vi "SR430.get bin width.vi"(0 "i ref in":refnum<vi>, 5 "error in (no error)":errorcluster) -> (14 "i ref out":refnum<vi>, 16 "binWidth [us]":dbl format="%.3f", 19 "error out":errorcluster)   [LabVIEW 2014, in "SR430.lvlib"]
doc: "reads the width of the bin from the unit."
uses:
  SR430.lvlib
  CSCore/CSApplicationBaseClasses/MCSBase/MCSBase.directionType.ctl
  CSCore/CSApplicationBaseClasses/MCSBase/MCSBase.serviceType.ctl
  CSlibraries/UtilityLib/UtilityLib.valueStatus.ctl
  CSCore/CSSystem/CoreDefs/CoreDefs.error_type.ctl
  CSinstr.lib/Sr430/SR430Driver.lvlib
  CSCore/CSSystem/CoreLib/CoreLib.lvlib
  CSCore/CSApplicationBaseClasses/MCSBase/MCSBase.lvlib
  CSlibraries/UtilityLib/UtilityLib.lvlib
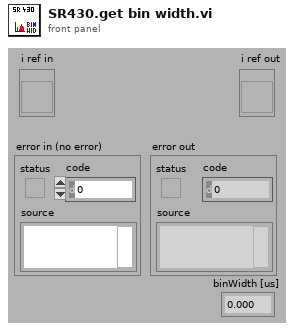
[diagram p1: front panel]
types:
  T1 = typedef "UtilityLib.lvlib/UtilityLib.valueStatus.ctl" = enum16{"no info available", "stand by/off", "on", "warning", "alarm/malfunction", "not implemented", "user action required", "important information", "system default", "control default", "indicator default", "button default"}
  T2 = typedef "MCSBase.lvlib/MCSBase.serviceType.ctl" = enum16{"counts", "totalCounts", "binWidth", "nOfBins", "nOfRecords", "status", "discrLevel", "discrSlope", "triggerLevel", "triggerSlope"}
  T3 = typedef "MCSBase.lvlib/MCSBase.directionType.ctl" = enum16{"unknown", "update actual value", "update nominal value", "update both"}
  T4 = typedef "CoreDefs.error_type.ctl" = enum16{"no error", "can't load process", "can't unload process", "process does not exist", "can't install process", "can't remove process", "unknown function", "time out", "can't execute function", "duplicate queue name", "super not found", "caller queue invalid", "can't ping process", "unknown error", "VISA Error", "VISA timeout", "GPIB timeout", "GPIB error", "communication error", "data type mismatch", "can't read data from OPC server", "can't write data to OPC server", "OET error", "function not implemented", "process already exists", "invalid Shared Variable name", "error writing Shared Variable", "error reading Shared Variable", "invalid client name", "corrupt database", "unknown class", "call not authorized", "parameter out of range", "OET timeout: can't get data to modify", "invalid queue name", "requested operation incompatible with current state", "event undefined", "event disabled", "state undefined", "caller is not a friend", "EventBuilder: bad eventID", "EventBuilder: no DAQ devices", "a thread must not stop itself", "UNUSED ELEMENT4", "DiscArchiver: eventData incomplete", "DiscArchiver: eventData does not belong to run", "DiscArchiver: can't open file", "DiscArchiver: can't write to file", "DiscArchiver: available disc space low", "can't acquire semaphore", "error reading data from database", "notifier object is not existing", "can't register process", "can't unregister process", "illegal event type", "object disabled", "object already exists", "can't change state", "Instrument not found", "no connection to remote node", "invalid reference", "N/A", "UNUSED ELEMENT 1", "element not found", "illegal TCP/IP connection detected", "object does not exist", "invalid access ID", "unknown CS system", "invalid privilige", "unsupported data type", "unsupported server type", "IO server already exists", "Shared Variable already exists"}
  T5 = typedef "SR430Driver.lvlib/SR430_VISA Control.ctl" = cluster{"VISA resource name":refnum<visa-resource-name>}
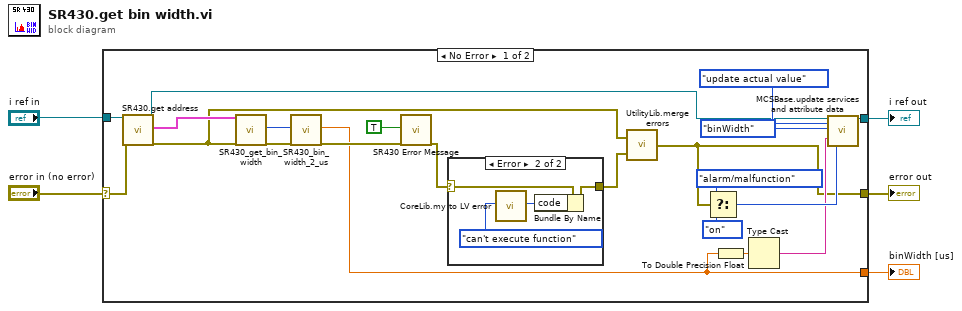
[diagram p0: block diagram]
diagram:
  n1 = case shown="No Error" "error in (no error)" {
    selector: "error in (no error)" -> [w17 w33]
    tunnel: "i ref in" -> [w26 w32]
    tunnel: [w6 w33] -> w4
    tunnel: [w8 w32] -> w3
    tunnel: [w7 _] -> w2
    frame No Error {
      n2 = call "SR430.get address.vi"("i ref in"=w26, "error in (no error)"=w17) -> ("i ref out"=w9:refnum<vi>, "address"=w25:T5, "error out"=w24:errorcluster)  [unwired: 15 in]
      n3 = call "SR430_get_bin_width.vi"("address"=w25, "error in (no error)"=w24) -> ("bin width"=w21:i32, "error out"=w22:errorcluster)  [unwired: 15 in, 1 out]
      n4 = call "SR430_bin_width_2_us.vi"("bin width"=w21, "error in (no error)"=w22) -> ("binWidth [us]"=w7:dbl, "error out"=w20:errorcluster)  [unwired: 15 in, 1 out]
      n5 = call "SR430 Error Message.vi"("addMessageToSource"=TRUE ("add message to source"), "error in (no error)"=w20) -> ("error out"=w23:errorcluster)  [unwired: 14 in, 3 out]
      n6 = case shown="Error" w23 {
        selector: w23 -> [w27 w31]
        tunnel: [w27 w28] -> w18
        frame No Error {
        }
        frame Error {
          n7 = call "CoreLib.my to LV error.vi"("ErrorTypes"=CoreDefs.error_type."can't execute function") -> ("LV error code"=w30:i32)  [unwired: 17 in, 1 out]
          n8 = Bundle By Name(cluster=w31, "code"=w30) -> (w28:errorcluster)
        }
      }
      n9 = call "UtilityLib.merge errors.vi"("error2 (no error)"=w18, "error1 (no error)"=w24) -> ("error out"=w6:errorcluster)
      n10 = Select(t=UtilityLib.valueStatus."alarm/malfunction" ("quality"), s=w6, f=UtilityLib.valueStatus."on") -> (s? t:f=w12:T1)
      n11 = To Double Precision Float(number=w7) -> (double precision float=w10:dbl)
      n12 = Type Cast(x=w10) -> (*(type *) &x=w11:string)  [unwired: 1 in]
      n13 = call "MCSBase.update services and attribute data.vi"("i ref in"=w9, "direction"=MCSBase.directionType."update actual value", "service"=MCSBase.serviceType."binWidth", "value"=w11, "quality"=w12) -> ("i ref out"=w8:refnum<vi>)  [unwired: 12 in, 2 out]
    }
    frame Error {
    }
  }
  "error out" <- w4
  "i ref out" <- w3
  "binWidth [us]" <- w2
